vi "Generate DIO Port Error.vi"(8 "Error in":errorcluster, 10 "DO Pins":u8[](array[numeric]), 11 "ChipKit Resource":T1) -> (0 "Error Out":errorcluster, 2 "DO Pins":u8[](array[numeric]), 3 "ChipKit Resource":T1={"COM Port"="", "Board Type"=enum."ChipKit uC32", "Connection Type"=enum."USB / Serial", "Baud Rate (115200)"=115200, "Bytes Per Packet (15)"=15, "DI Port Num Pins"=0, "DO Port Num Pins"=0})   [LabVIEW 2011, in "LabVIEW Interface for ChipKit.lvlib"]
uses:
  LabVIEW Interface for ChipKit.lvlib
  Type Defs/Chipkit Resource.ctl
  Type Defs/Board Type.ctl
  Type Defs/Connection Type.ctl
  Type Defs/Pin Type.ctl
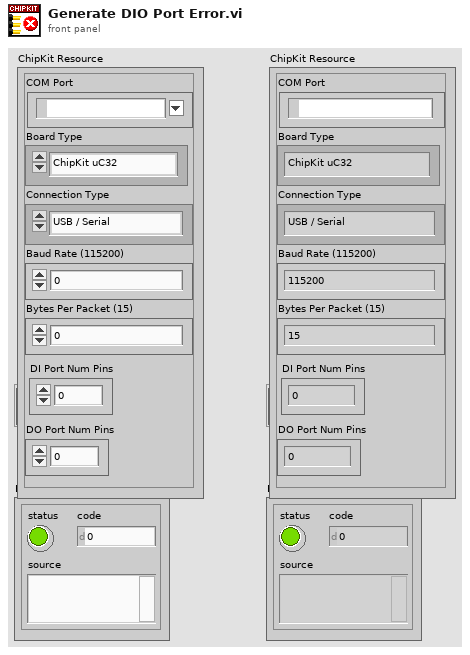
[diagram p1: front panel]
types:
  T1 = typedef "LabVIEW Interface for ChipKit.lvlib/Chipkit Resource.ctl" = cluster{"COM Port":refnum<visa-resource-name>, "Board Type":T2, "Connection Type":T3, "Baud Rate (115200)":u32, "Bytes Per Packet (15)":u32, "DI Port Num Pins":i32, "DO Port Num Pins":i32}
  T2 = typedef "LabVIEW Interface for ChipKit.lvlib/Board Type.ctl" = enum16{"ChipKit uC32", "ChipKit Uno32", "ChipKit Max32"}
  T3 = typedef "LabVIEW Interface for ChipKit.lvlib/Connection Type.ctl" = enum8{"USB / Serial", "XBEE", "BlueSmirf (Bluetooth)"}
  T4 = typedef "LabVIEW Interface for ChipKit.lvlib/Pin Type.ctl" = enum8{"Analog", "Digital", "PWM", "Tone"}
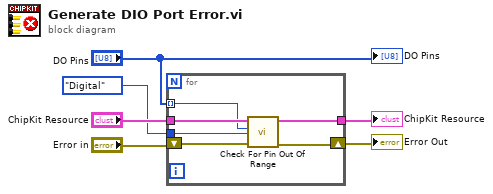
[diagram p0: block diagram]
diagram:
  n1 = for {
    tunnel: "DO Pins" -> [w8] mode=indexing
    shift-right: [w11] -> w6
    shift-left: "Error in" -> [w12]
    tunnel: "ChipKit Resource" -> [w10]
    tunnel: [w9] -> w2
    tunnel: Pin_Type."Digital" ("Pin Type") -> [w7]
    n2 = call "Check For Pin Out Of Range.vi"("Error In"=w12, "Pin Type"=w7, "User Pin Number"=w8, "Arduino Resource"=w10) -> ("Error Out"=w11:errorcluster, "Arduino Resource"=w9:T1)  [unwired: 6 in]
  }
  "Error Out" <- w6
  "ChipKit Resource" <- w2
  "DO Pins" <- "DO Pins"
